vi "THD_Harmonics.vi"() -> ()   [LabVIEW 2015]
panel:
  out "Specific Harmonic":i32
  out "SINAD":i32
  out "THD":i32
  out "Peak to Peak":i32
  out "RMS":i32
  out "Waveform Graph":dynamicdata(graph)
  in  "Frequency":i32
  in  "Voltage Source":i32
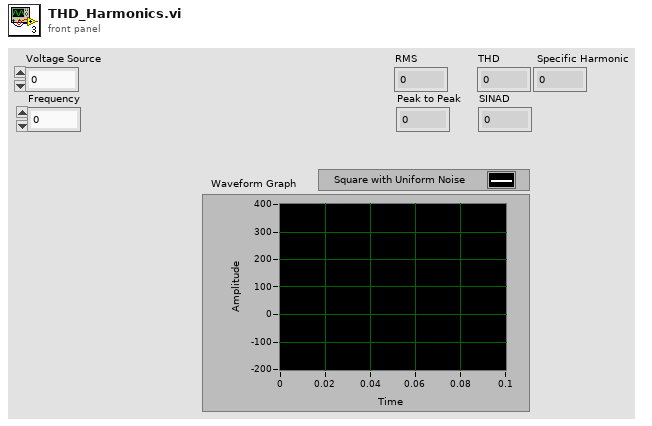
[diagram p1: front panel]
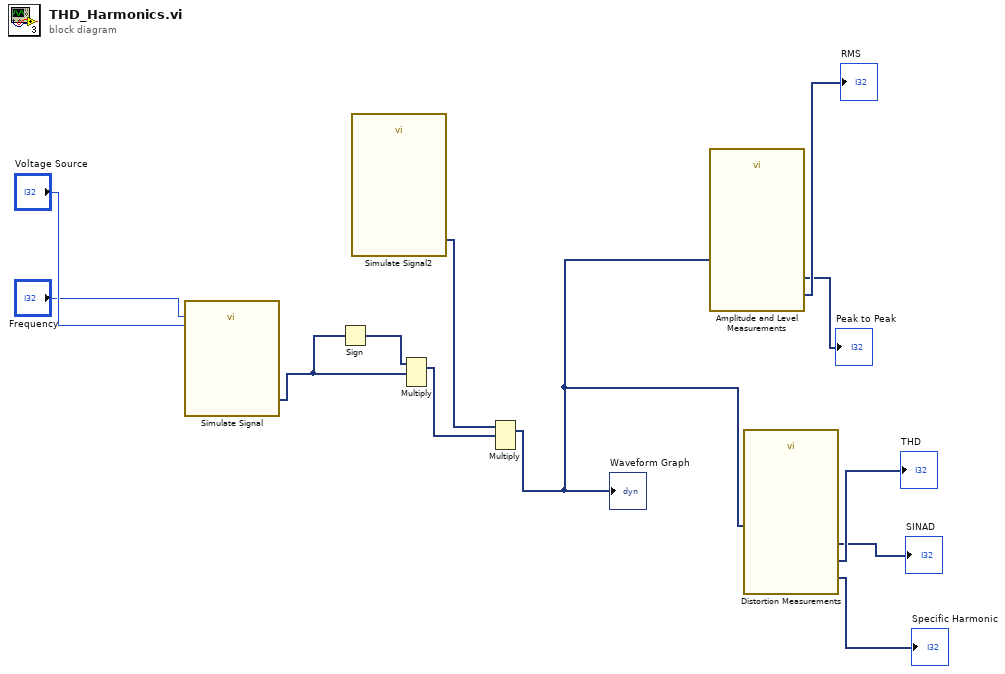
[diagram p0: block diagram]
diagram:
  n1 = call "Simulate Signal"("Frequency"="Frequency", "Amplitude"="Voltage Source") -> ("Sine"=w10:dynamicdata)  [unwired: 12 in, 1 out]
  n2 = Sign(1:w10) -> (0:w9:dynamicdata)
  n3 = call "Simulate Signal2"() -> ("Square with Uniform Noise"=w7:dynamicdata)  [unwired: 14 in, 1 out]
  n4 = Multiply(1:w10, 2:w9) -> (0:w8:dynamicdata)  [unwired: 1 in, 1 out]
  n5 = Multiply(1:w8, 2:w7) -> (0:w3:dynamicdata)  [unwired: 1 in, 1 out]
  "Waveform Graph" <- w3
  n6 = call "Amplitude and Level Measurements"("Signals"=w3) -> ("RMS"=→"RMS":dynamicdata, "Peak to Peak"=→"Peak to Peak":dynamicdata)  [unwired: 12 in, 1 out]
  n7 = call "Distortion Measurements"("Signals"=w3) -> ("SINAD (dB)"=→"SINAD":dynamicdata, "Specific Harmonic"=→"Specific Harmonic":dynamicdata, "THD"=→"THD":dynamicdata)  [unwired: 7 in, 1 out]
